vi "GetQ.vi"(8 "error in (no error)":errorcluster, 11 "Mode (Get)":enum16{"Get", "Close", "Init"}(ring)) -> (0 "error out":errorcluster, 3 "Q out":refnum<queue>)   [LabVIEW 2017, in "Error.lvlib"]
doc: "Maintains the Q refferance for the module's main coms"
uses:
  Error.lvlib
  ctl/MainData.ctl
  ctl/MainStates.ctl
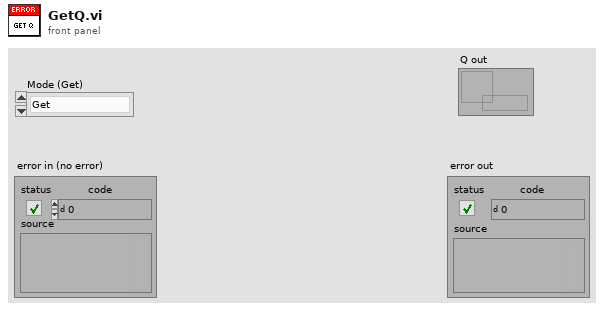
[diagram p1: front panel]
types:
  T1 = typedef "Error.lvlib/MainData.ctl" = cluster{"State":T2, "Variant":variant}
  T2 = typedef "Error.lvlib/MainStates.ctl" = enum16{"Timeout", "Error", "Exit", "Init", "ClassError", "LogError", "Shutdown", "Warning"}
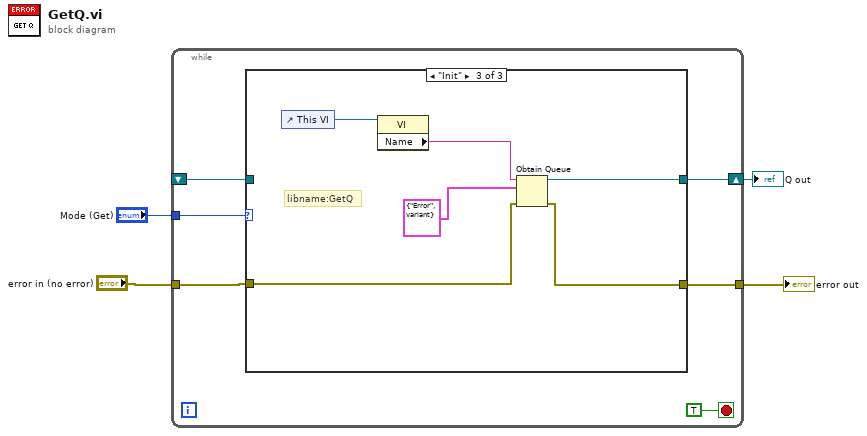
[diagram p0: block diagram]
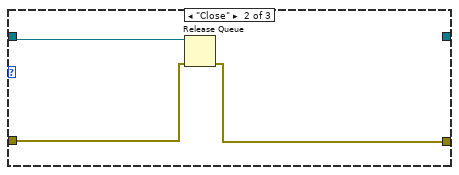
[diagram p3: hidden frame]
diagram:
  n1 = while {
    tunnel: "Mode (Get)" -> [w9]
    tunnel: "error in (no error)" -> [w8]
    tunnel: [w7] -> w2
    shift-right: [w6] -> w1
    shift-left: _ -> [w5]
    stop <- TRUE stop-if-true
    n2 = case shown="\"Init\"" w9 {
      tunnel: w8 -> [w11 w14 w19]
      tunnel: [w11 w13 w18] -> w7
      tunnel: [w12 _ w17] -> w6
      tunnel: w5 -> [w12 w15 _]
      frame "Get", Default {
      }
      frame "Close" {
        n3 = Release Queue(queue=w15, error in (no error)=w14) -> (error out=w13:errorcluster)  [unwired: 1 in, 2 out]
      }
      frame "Init" {
        # "libname:GetQ"
        n4 = control-ref of="This VI"() -> (w21:refnum<vi>)
        n5 = property class="VI"(reference=w21) -> ("Name"=w20:string)  [unwired: 1 in, 2 out]
        n6 = Obtain Queue(name (unnamed)=w20, element data type=T1 {"State"=enum."Error", "Variant"=variant} ("Data"), error in (no error)=w19) -> (queue out=w17:refnum<queue>, error out=w18:errorcluster)  [unwired: 2 in, 1 out]
      }
    }
  }
  "error out" <- w2
  "Q out" <- w1
